vi "closeHDF5.vi"(8 "error in (no error)":errorcluster, 11 "Imaging in":refnum<class "Imaging.lvclass">) -> (0 "error out":errorcluster, 3 "Imaging out":refnum<class "Imaging.lvclass">)   [LabVIEW 2014, in "Imaging.lvclass"]
uses:
  Imaging.lvclass
  Imaging.lvclass/Imaging.ctl
  private/HDF5Tools32/LabView/HDF5Tools.lvlib
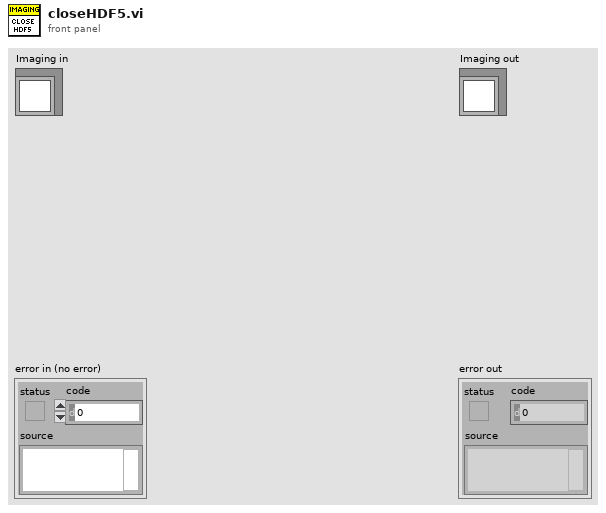
[diagram p1: front panel]
types:
  T1 = typedef "AviRefnum.ctl" = refnum<k1>
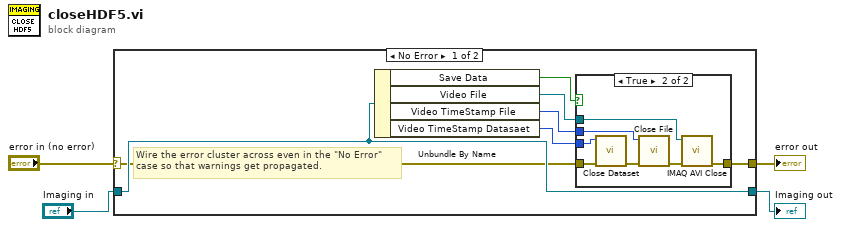
[diagram p0: block diagram]
diagram:
  n1 = case shown="No Error" "error in (no error)" {
    selector: "error in (no error)" -> [w7 w21]
    tunnel: [w6 w21] -> w3
    tunnel: [w11 w20] -> w1
    tunnel: "Imaging in" -> [w11 w20]
    frame No Error {
      # "Wire the error cluster across even in the \"No Error\"\ncase so that warnings get propagated."
      n2 = Unbundle By Name(w11) -> ("Save Data"=w5:bool, "Video File"=w8:T1, "Video TimeStamp File"=w9:i32, "Video TimeStamp Datasaet"=w10:i32)
      n3 = case shown="True" w5 {
        tunnel: w10 -> [_ w18]
        tunnel: w9 -> [_ w17]
        tunnel: [w12 w15] -> w6
        tunnel: w8 -> [_ w14]
        tunnel: w7 -> [w12 w13]
        frame False {
        }
        frame True {
          n4 = call "Close Dataset.vi"("error in (no error)"=w13, "dataset_id"=w18) -> ("error out"=w19:errorcluster)  [unwired: 9 in]
          n5 = call "Close File.vi"("error in (no error)"=w19, "file_id"=w17) -> ("error out"=w16:errorcluster)  [unwired: 9 in]
          n6 = call "IMAQ AVI Close"("error in (no error)"=w16, "Avi Refnum"=w14) -> ("error out"=w15:errorcluster)  [unwired: 9 out]
        }
      }
    }
    frame Error {
    }
  }
  "error out" <- w3
  "Imaging out" <- w1
